vi "Test-Tracer-Virtual.vi"() -> ()   [LabVIEW 2013]
uses:
  Robot/Virtual Systems/Tracer-V/Tracer-V.lvclass
  Robot/Logical Systems/TraceMessage/Trace.lvclass
  <vilib>/ActorFramework/Message Queue/Message Queue.lvclass/Message Queue.ctl
  Robot/Logical Systems/XBoxController/XBoxController.lvclass
  Robot/Logical Systems/Tracer Messages/Record TraceMessage Msg/Log Trace Msg.lvclass/Log Trace Msg.ctl
  <vilib>/ActorFramework/Message Enqueuer/Message Enqueuer.lvclass/Message Enqueuer.ctl
  <vilib>/ActorFramework/Message Enqueuer/Enqueue.vi
  <vilib>/ActorFramework/Message Priority Queue/Priority Enqueue.vi
  Robot/Logical Systems/Tracer Messages/Record TraceMessage Msg/Log Trace Msg.lvclass
  <vilib>/ActorFramework/Stop Msg/Stop Msg.lvclass
  <vilib>/ActorFramework/Message Queue/Message Queue.lvclass
  <vilib>/ActorFramework/Actor/Actor.lvclass
panel:
  out "Message To Queu":string
  out "XBox Controller Layout":T1 {"Right Joystick Right" scale=-1.0..1.0; "Left Joystick Right" scale=-1.0..1.0; "Right Joystick Forward" scale=-1.0..1.0; "Left Joystick Forward" scale=-1.0..1.0}
  out "FlattenType":string
  out "Flattened":string
  in  "milliseconds to wait - DeQUe":u32=1000 step=10
  out "# elements in queue":i32
  out "Last Message":string
  in  "milliseconds to wait":u32=1000 step=10
  in  "stop":bool
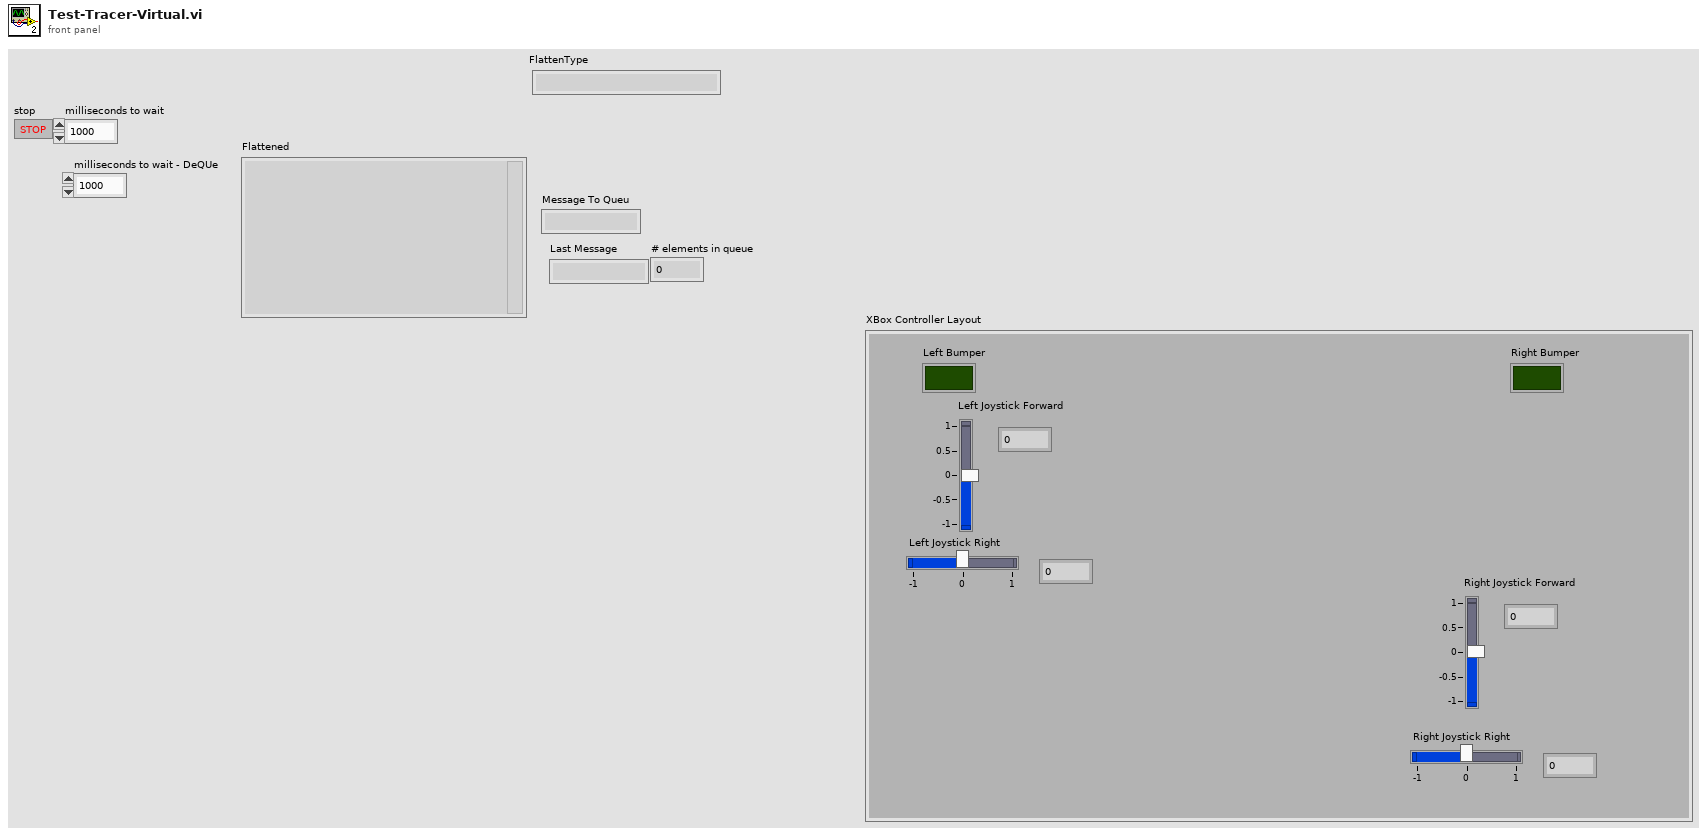
[diagram p1: front panel]
types:
  T1 = cluster{"Left Bumper":bool, "Right Bumper":bool, "Left Joystick Forward":dbl, "Left Joystick Right":dbl, "Right Joystick Forward":dbl, "Right Joystick Right":dbl}
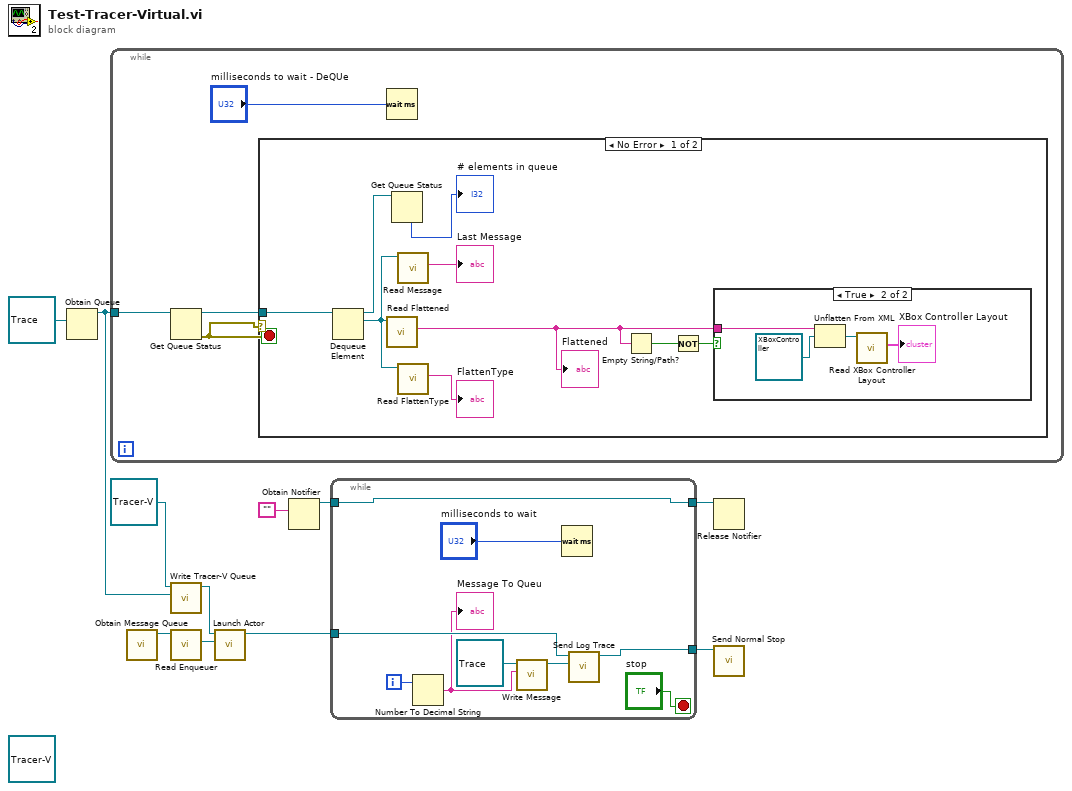
[diagram p0: block diagram]
diagram:
  (unwired) refnum<class "Tracer-V.lvclass"> refnum ("Tracer-V.lvclass")
  n1 = Obtain Queue(element data type=refnum<class "Trace.lvclass"> refnum ("Trace.lvclass")) -> (queue out=w1:refnum<queue>)  [unwired: 4 in, 2 out]
  n2 = while {
    tunnel: w1 -> [w14]
    stop <- w13 stop-if-true
    n3 = Get Queue Status(queue=w14) -> (queue out=w12:refnum<queue>, error out=w13:errorcluster)  [unwired: 2 in, 6 out]
    n4 = case shown="No Error" w13 {
      tunnel: w12 -> [w22 _]
      frame No Error {
        n5 = Dequeue Element(queue=w22) -> (queue out=w17:refnum<queue>, element=w21:refnum<class "Trace.lvclass">)  [unwired: 2 in, 2 out]
        n6 = call-dynamic "Read Flattened.vi"("TraceMessage in"=w21) -> ("Flattened"=w19:string)  [unwired: 8 in, 2 out]
        "Flattened" <- w19
        n7 = Get Queue Status(queue=w17) -> (# elements in queue=→"# elements in queue":i32)  [unwired: 2 in, 7 out]
        n8 = call-dynamic "Read Message.vi"("TraceMessage in"=w21) -> ("Message"=→"Last Message":string)  [unwired: 8 in, 2 out]
        n9 = call-dynamic "Read FlattenType.vi"("TraceMessage in"=w21) -> ("FlattenType"=→"FlattenType":string)  [unwired: 8 in, 2 out]
        n10 = Empty String/Path?(string/path=w19) -> (empty?=w20:bool)
        n11 = Not(x=w20) -> (.not. x?=w18:bool)
        n12 = case shown="True" w18 {
          tunnel: w19 -> [_ w28]
          frame False {
          }
          frame True {
            n13 = Unflatten From XML(xml string=w28, type=refnum<class "XBoxController.lvclass"> refnum ("XBoxController.lvclass")) -> (value=w26:refnum<class "XBoxController.lvclass">)  [unwired: 1 in, 1 out]
            n14 = call-dynamic "Read XBox Controller Layout.vi"("XBoxController in"=w26) -> ("XBox Controller Layout"=→"XBox Controller Layout":T1)  [unwired: 8 in, 2 out]
          }
        }
      }
      frame Error {
      }
    }
    n15 = Wait (ms)(milliseconds to wait="milliseconds to wait - DeQUe") -> ()  [unwired: 1 out]
  }
  n16 = call <vilib>:"Obtain Message Queue.vi"() -> ("Message Queue"=w11:refnum<class "Message Queue.lvclass">)  [unwired: 10 in, 1 out]
  n17 = call-dynamic "Write Tracer-V Queue.vi"("TraceMessage Queue"=w1, "Tracer-V in"=refnum<class "Tracer-V.lvclass"> refnum ("Tracer-V.lvclass")) -> ("Tracer-V out"=w2:refnum<class "Tracer-V.lvclass">)  [unwired: 8 in, 1 out]
  n18 = call <vilib>:"Read Enqueuer.vi"("Message Queue"=w11) -> ("Message Enqueuer"=w10:refnum<class "Message Enqueuer.lvclass">)  [unwired: 10 in]
  n19 = call <vilib>:"Launch Actor.vi"("Actor-to-Caller Enqueuer"=w10, "Actor"=w2) -> ("Caller-To-Actor Enqueuer"=w5:refnum<class "Message Enqueuer.lvclass">)  [unwired: 8 in, 1 out]
  n20 = Obtain Notifier(notification data type="") -> (notifier out=w8:refnum<notifier>)  [unwired: 3 in, 2 out]
  n21 = while {
    tunnel: w5 -> [w34]
    tunnel: [w33] -> w9
    tunnel: w8 -> [w35]
    tunnel: [w35] -> w6
    i -> [w30]
    stop <- "stop" stop-if-true
    n22 = Number To Decimal String(number=w30) -> (decimal integer string=w29:string)  [unwired: 1 in]
    "Message To Queu" <- w29
    n23 = call-dynamic "Write Message.vi"("Message"=w29, "TraceMessage in"=refnum<class "Trace.lvclass"> refnum ("Trace.lvclass")) -> ("TraceMessage out"=w31:refnum<class "Trace.lvclass">)  [unwired: 8 in, 1 out]
    n24 = Wait (ms)(milliseconds to wait="milliseconds to wait") -> ()  [unwired: 1 out]
    n25 = call "Send Log Trace.vi"("TraceMessage.lvclass"=w31, "Message Enqueuer"=w34) -> ("Message Enqueuer out"=w33:refnum<class "Message Enqueuer.lvclass">)  [unwired: 8 in, 1 out]
  }
  n26 = Release Notifier(notifier=w6) -> ()  [unwired: 2 in, 3 out]
  n27 = call <vilib>:"Send Normal Stop.vi"("Message Enqueuer"=w9) -> ()  [unwired: 10 in, 1 out]
